vi "array_max.vi"() -> ()   [LabVIEW 2021]
uses:
  <vilib>/numeric/Random Number (Range) DBL.vi
panel:
  out "Index of Max":dbl
  out "Maximum value":dbl
  out "Array":dbl[](array[numeric])
  out "Done":bool
  out "random number":dbl
  out "iteration counter":i32
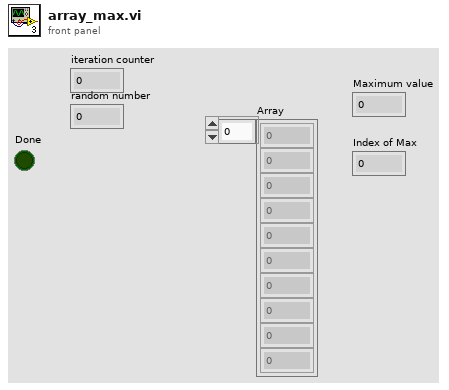
[diagram p1: front panel]
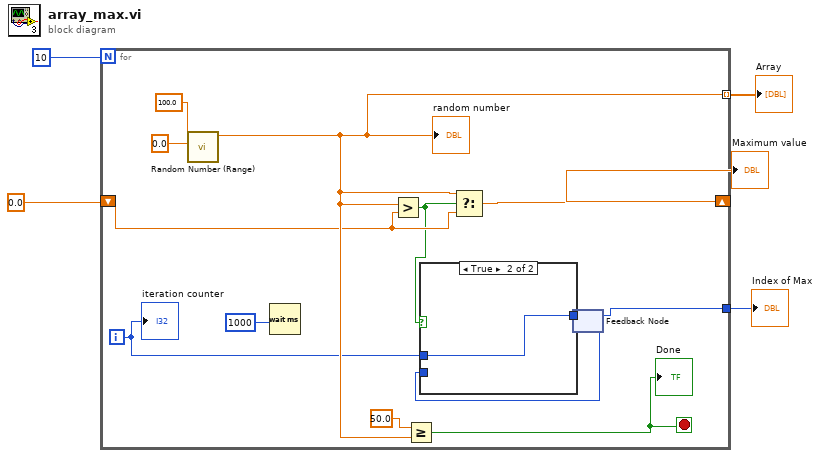
[diagram p0: block diagram]
diagram:
  n1 = for {
    N: 10 -> [_]
    tunnel: [w12] -> w4 mode=indexing
    shift-right: [w11] -> w3
    shift-left: 0.0 -> [w10]
    tunnel: [w6] -> w1
    i -> [w8]
    stop <- w13 stop-if-true
    n2 = call-poly <vilib>:"Random Number (Range).vi"("lower bound (0)"=0.0, "upper bound (100)"=100.0) -> ("number"=w12:dbl)  [unwired: 9 in]
    "random number" <- w12
    n3 = Wait (ms)(milliseconds to wait=1000) -> ()  [unwired: 1 out]
    n4 = Greater?(x=w12, y=w10) -> (0:w9:bool)
    n5 = Greater Or Equal?(x=50.0, y=w12) -> (x >= y?=w13:bool)
    "Done" <- w13
    n6 = Select(t=w12, s=w9, f=w10) -> (s? t:f=w11:dbl)
    n7 = feedback #1() -> (w6:i32)  [unwired: 1 in]
    n8 = case shown="True" w9 {
      tunnel: [w18 w19] -> w7
      tunnel: w8 -> [_ w19]
      tunnel: w6 -> [w18 _]
      frame False {
      }
      frame True {
      }
    }
    n9 = feedback-in #1(w7) -> ()
    "iteration counter" <- w8
  }
  "Array" <- w4
  "Maximum value" <- w3
  "Index of Max" <- w1
